vi "datei schicken.vi"   [LabVIEW 2010]
uses:
  <vilib>/addons/internet/NI_InternetTK_FTP_VIs.lvlib
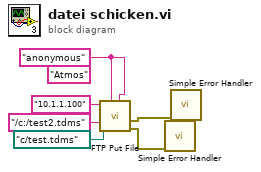
[diagram p0: block diagram]
diagram:
  w1 = "anonymous" ("user")
  (unwired) "Atmos" ("user")
  n1 = call <vilib>:"FTP Put File.vi"("password"=w1, "user"=w1, "local path"=path "c:/test.tdms", "remote path"="/c:/test2.tdms", "host"="10.1.1.100") -> ("error out"=w2:errorcluster, "file error"=w3:errorcluster)  [unwired: 5 in]
  n2 = call <vilib>:"Simple Error Handler.vi"("error in (no error)"=w2) -> ()  [unwired: 4 in, 5 out]
  n3 = call <vilib>:"Simple Error Handler.vi"("error in (no error)"=w3) -> ()  [unwired: 4 in, 5 out]
